vi "Write Input Registers.vi"(8 "error in (no error)":errorcluster, 9 "register values":u16[](array[numeric]), 10 "starting address":u16, 11 "Standard Data Model in":refnum<class "Standard Data Model.lvclass">) -> (0 "error out":errorcluster, 3 "Standard Data Model out":refnum<class "Standard Data Model.lvclass">)   [LabVIEW 2021, in "Standard Data Model.lvclass"]
doc: "Writes the values of multiple input register values in series, starting at address M."
uses:
  Standard Data Model.lvclass
  Standard Data Model.lvclass/Standard Data Model.ctl
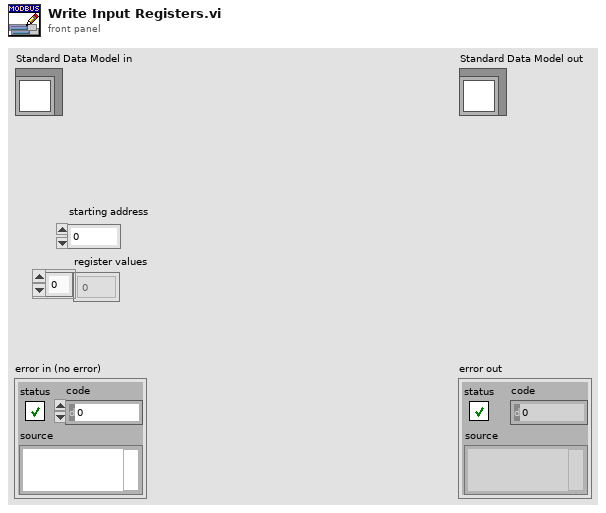
[diagram p1: front panel]
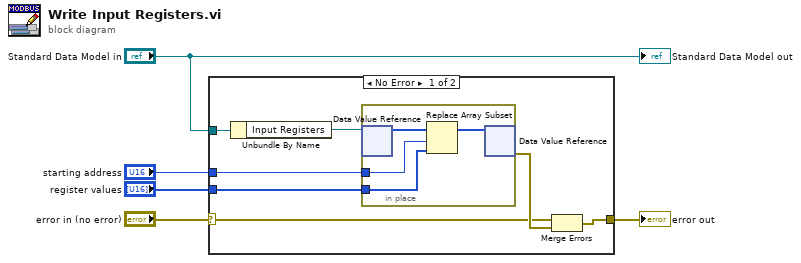
[diagram p0: block diagram]
diagram:
  n1 = case shown="No Error" "error in (no error)" {
    selector: "error in (no error)" -> [w6 w17]
    tunnel: "starting address" -> [w12 _]
    tunnel: "register values" -> [w11 _]
    tunnel: "Standard Data Model in" -> [w10 _]
    tunnel: [w8 w17] -> w2
    frame No Error {
      n2 = Unbundle By Name(w10) -> ("Input Registers"=w9:refnum<data-value>)
      n3 = in-place {
        in-place-border: w12 -> [w16]
        in-place-border: w11 -> [w15]
        n4 = in-place-dvr #1(w9) -> (w14:u16[])  [unwired: 1 out]
        n5 = Replace Array Subset(array=w14, new element=w15, index=w16) -> (w13:u16[])
        n6 = in-place-dvr #1(w13) -> (w7:errorcluster)  [unwired: 1 out]
      }
      n7 = Merge Errors(w6, w7) -> (w8:errorcluster)
    }
    frame Error {
    }
  }
  "error out" <- w2
  "Standard Data Model out" <- "Standard Data Model in"
